vi "rad_Configure App Images Settings Dialog.vi"(8 "error in (no error)":errorcluster, 11 "App Images Settings":T1) -> (0 "error out":errorcluster, 1 "Cancelled":bool, 3 "App Images Settings":T1)   [LabVIEW 2013]
uses:
  TypeDefs/rad_App Images Settings.ctl
  Util/FP Control/FP Control Functions.ctl
panel:
  in  "Application Image Repository":path
  in  "Cancel":bool
  in  "OK":bool
  # "Application Images Settings"
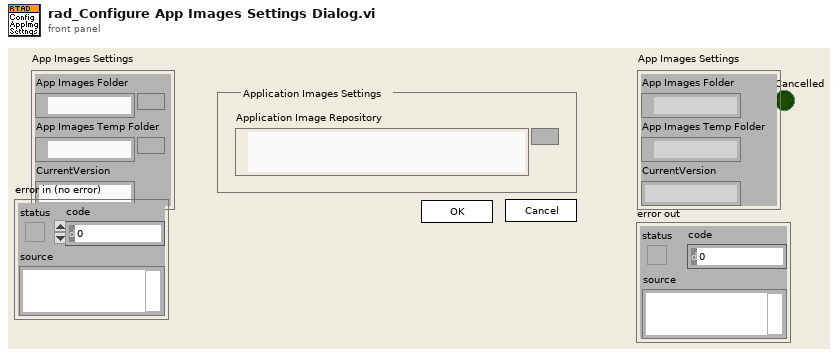
[diagram p1: front panel]
types:
  T1 = typedef "rad_App Images Settings.ctl" = cluster{"App Images Folder":path, "App Images Temp Folder":path, "CurrentVersion":string}
  T2 = typedef "FP Control Functions.ctl" = enum16{"Open", "Close", "Bring To Front", "Center"}
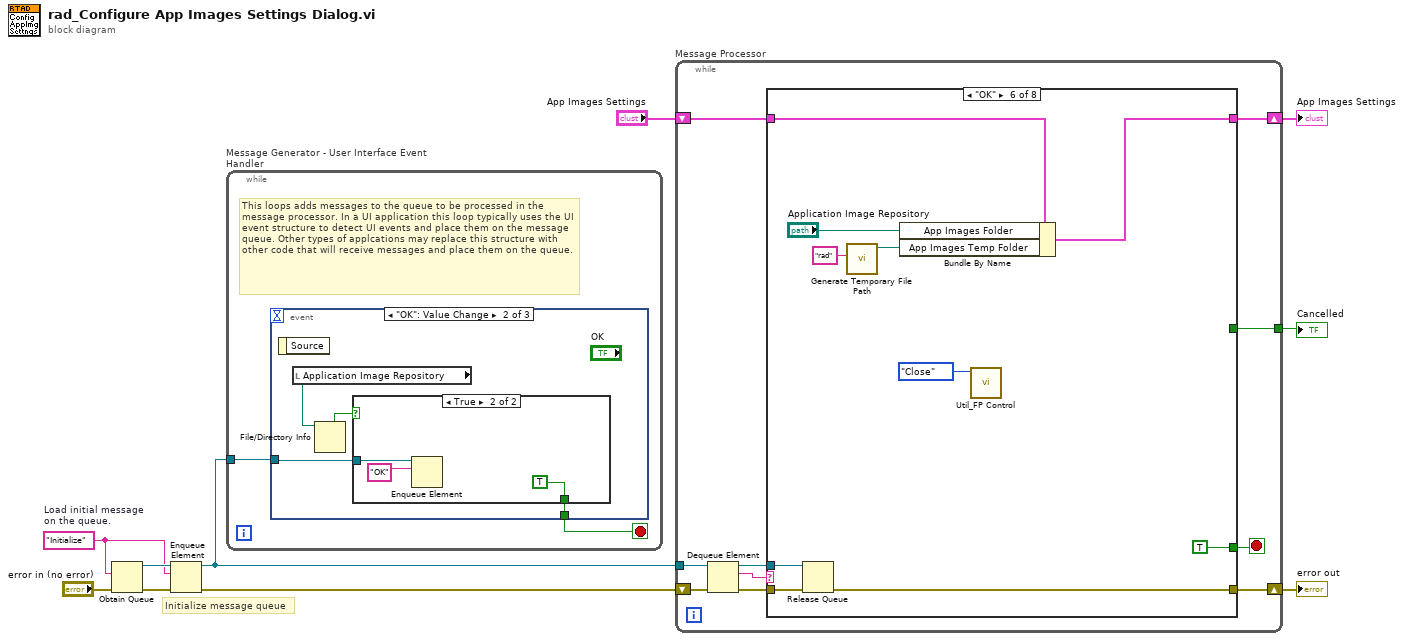
[diagram p0: block diagram]
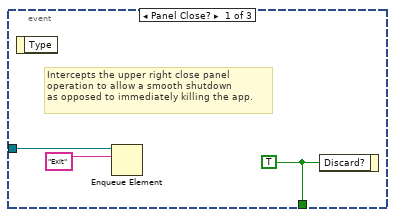
[diagram p2: hidden frame]
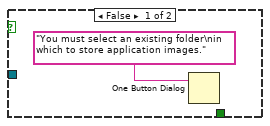
[diagram p3: hidden frame]
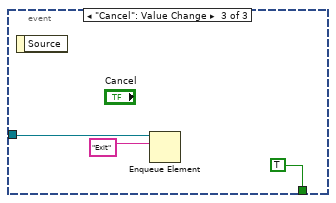
[diagram p4: hidden frame]
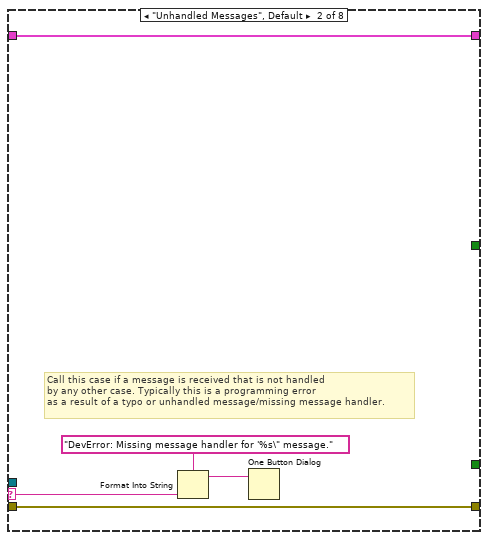
[diagram p6: hidden frame]
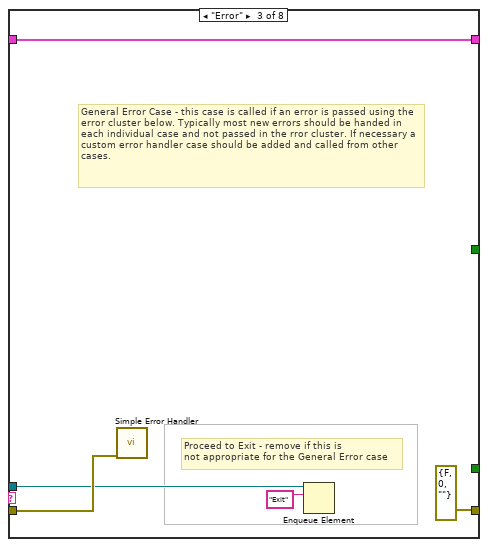
[diagram p7: hidden frame]
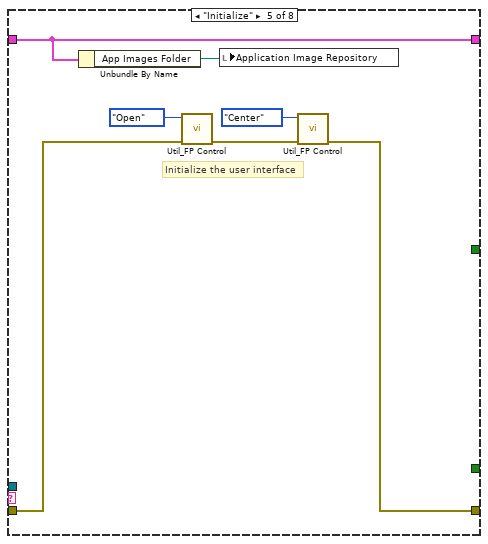
[diagram p9: hidden frame]
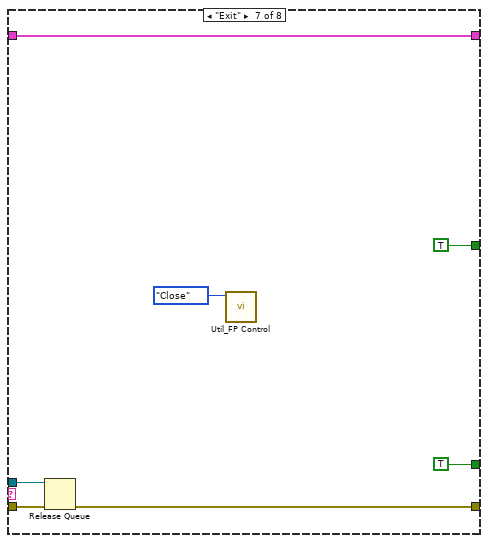
[diagram p10: hidden frame]
diagram:
  w2 = "Initialize"  # Load initial message on the queue.
  # "Initialize message queue"
  n1 = Obtain Queue(element data type=w2, error in (no error)="error in (no error)") -> (queue out=w3:refnum<queue>, error out=w10:errorcluster)  [unwired: 3 in, 1 out]
  n2 = Enqueue Element(queue=w3, element=w2, error in (no error)=w10) -> (queue out=w1:refnum<queue>, error out=w4:errorcluster)  [unwired: 1 in, 1 out]
  n3 = while "Message Generator - User Interface Event Handler" {
    tunnel: w1 -> [w11]
    stop <- w12 stop-if-true
    # "This loops adds messages to the queue to be processed in the message processor. In a UI application this loop typically uses the UI event structure to detect UI events and place them on the message queue. Other types of applcations may replace this structure with other code that will receive messages and place them on the queue."
    n4 = event shown="[1] \"OK\": Value Change" {
      selector: _ -> [_ _ _]
      dyn-events: _ -> [_ _ _]
      timeout: _ -> [_ _ _]
      tunnel: [w15 w18 TRUE ("Discard?")] -> w12
      tunnel: w11 -> [w14 w19 w26]
      event Panel Close? {
        w15 = TRUE ("Discard?")
        # "Intercepts the upper right close panel\noperation to allow a smooth shutdown\nas opposed to immediately killing the app."
        n5 = event-data() -> ()  [unwired: 2 out]
        n6 = Enqueue Element(queue=w14, element="Exit") -> ()  [unwired: 2 in, 3 out]
        n7 = event-data("Discard?"=w15) -> ()  [unwired: 1 in, 1 out]
      }
      event "OK": Value Change {
        n8 = event-data() -> ()  [unwired: 2 out]
        n9 = local read "Application Image Repository"() -> (w17:path)
        n10 = File/Directory Info(path=w17) -> (directory=w16:bool)  [unwired: 1 in, 6 out]
        n11 = case shown="True" w16 {
          tunnel: w19 -> [_ w23]
          tunnel: [_ TRUE ("Discard?")] -> w18
          frame False {
            n12 = One Button Dialog(message="You must select an existing folder\nin which to store application images.") -> ()  [unwired: 1 in, 1 out]
          }
          frame True {
            n13 = Enqueue Element(queue=w23, element="OK") -> ()  [unwired: 2 in, 3 out]
          }
        }
      }
      event "Cancel": Value Change {
        n14 = event-data() -> ()  [unwired: 2 out]
        n15 = Enqueue Element(queue=w26, element="Exit") -> ()  [unwired: 2 in, 3 out]
      }
    }
  }
  n16 = while "Message Processor" {
    shift-left: w4 -> [w33]
    shift-right: [w34] -> w5
    tunnel: w1 -> [w32]
    shift-right: [w29] -> w8
    shift-left: "App Images Settings" -> [w30]
    tunnel: [w28] -> w7
    stop <- w27 stop-if-true
    n17 = Dequeue Element(queue=w32, error in (no error)=w33) -> (queue out=w36:refnum<queue>, element=w31:string, error out=w35:errorcluster)  [unwired: 1 in, 1 out]
    n18 = case shown="\"OK\"" w31 {
      selector: w31 -> [_ w42 _ _ _ _ _ _]
      tunnel: w36 -> [_ _ w46 _ _ w66 w73 _]
      tunnel: w35 -> [w38 w43 w47 w49 w52 w67 w74 w75]
      tunnel: [w38 w43 errorcluster {"status"=FALSE, "code"=0, "source"=""} ("error out") w49 w51 w65 w72 w75] -> w34
      tunnel: w30 -> [w37 w39 w44 w50 w56 w64 w71 w76]
      tunnel: [w37 w39 w44 w50 w56 w63 w71 w76] -> w29
      tunnel: [_ _ _ _ _ _ TRUE _] -> w28
      tunnel: [_ _ _ _ _ TRUE TRUE _] -> w27
      frame "", "Wait" {
      }
      frame "Unhandled Messages", Default {
        # "Call this case if a message is received that is not handled \nby any other case. Typically this is a programming error\nas a result of a typo or unhandled message/missing message handler."
        n19 = Format Into String(format string="DevError: Missing message handler for '%s\" message." ("message"), w42) -> (resulting string=w40:string)  [unwired: 2 in, 1 out]
        n20 = One Button Dialog(message=w40) -> ()  [unwired: 2 out]
      }
      frame "Error" {
        # "Proceed to Exit - remove if this is\nnot appropriate for the General Error case"
        # "General Error Case - this case is called if an error is passed using the error cluster below. Typically most new errors should be handed in each individual case and not passed in the rror cluster. If necessary a custom error handler case should be added and called from other cases."
        n21 = call <vilib>:"Simple Error Handler.vi"("error in (no error)"=w47) -> ()  [unwired: 1 in, 8 out]
        n22 = Enqueue Element(queue=w46, element="Exit") -> ()  [unwired: 2 in, 3 out]
      }
      frame "*** Dialog Operations ***" {
      }
      frame "Initialize" {
        # "Initialize the user interface"
        n23 = Unbundle By Name(w56) -> ("App Images Folder"=w55:path)
        n24 = call "Util_FP Control.vi"("error in (no error)"=w52, "Function"=FP_Control_Functions."Open") -> ("error out"=w53:errorcluster)  [unwired: 9 out]
        n25 = local write "Application Image Repository"(w55) -> ()
        n26 = call "Util_FP Control.vi"("error in (no error)"=w53, "Function"=FP_Control_Functions."Center") -> ("error out"=w51:errorcluster)  [unwired: 9 out]
      }
      frame "OK" {
        n27 = Release Queue(queue=w66, error in (no error)=w67) -> (error out=w65:errorcluster)  [unwired: 1 in, 2 out]
        n28 = call <vilib>:"Generate Temporary File Path.vi"("Temporary File Extension (tmp)"="rad") -> ("Unique Temporary File Path"=w59:path)  [unwired: 9 in, 1 out]
        n29 = Bundle By Name(cluster=w64, "App Images Folder"="Application Image Repository", "App Images Temp Folder"=w59) -> (w63:T1)
        n30 = call "Util_FP Control.vi"("Function"=FP_Control_Functions."Close") -> ()  [unwired: 1 in, 10 out]
      }
      frame "Exit" {
        n31 = Release Queue(queue=w73, error in (no error)=w74) -> (error out=w72:errorcluster)  [unwired: 1 in, 2 out]
        n32 = call "Util_FP Control.vi"("Function"=FP_Control_Functions."Close") -> ()  [unwired: 1 in, 10 out]
      }
      frame "*** Other Operations ***" {
      }
    }
  }
  "App Images Settings" <- w8
  "Cancelled" <- w7
  "error out" <- w5
